vi "Character Status.vi"(4 "Character":string) -> (7 "Status":T1=enum."Unmodified")   [LabVIEW 2020, in "VolatusGUI.lvlib" / "Git Updater Module.lvclass"]
uses:
  Git Updater Module.lvclass
  Git Updater Module.lvclass/Git Updater Module.ctl
  Status.ctl
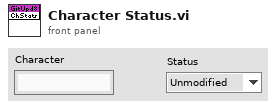
[diagram p1: front panel]
types:
  T1 = typedef "VolatusGUI.lvlib/Git Updater Module.lvclass/Status.ctl" = enum16{"UNKNOWN", "Unmodified", "Modified", "Added", "Deleted", "Renamed", "Unmerged", "Untracked", "Ignored"}
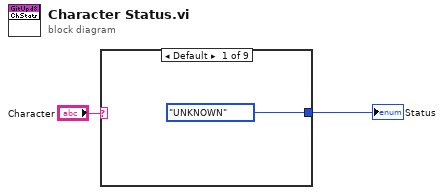
[diagram p0: block diagram]
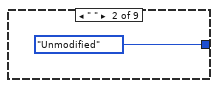
[diagram p2: hidden frame]
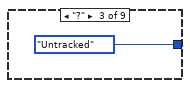
[diagram p3: hidden frame]
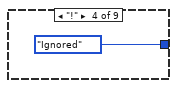
[diagram p4: hidden frame]
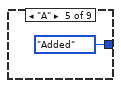
[diagram p5: hidden frame]
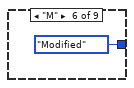
[diagram p6: hidden frame]
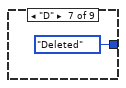
[diagram p7: hidden frame]
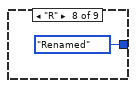
[diagram p8: hidden frame]
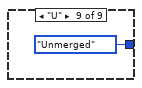
[diagram p9: hidden frame]
diagram:
  n1 = case shown="Default" "Character" {
    tunnel: [Status."UNKNOWN" ("Status") Status."Unmodified" ("Status") Status."Untracked" ("Status") Status."Ignored" ("Status") Status."Added" ("Status") Status."Modified" ("Status") Status."Deleted" ("Status") Status."Renamed" ("Status") Status."Unmerged" ("Status")] -> w1
    frame Default {
    }
    frame " " {
    }
    frame "?" {
    }
    frame "!" {
    }
    frame "A" {
    }
    frame "M" {
    }
    frame "D" {
    }
    frame "R" {
    }
    frame "U" {
    }
  }
  "Status" <- w1
